vi "runBraking.vi"(6 "Fault?":bool, 7 "x acceleration":dbl, 8 "error in (no error)":errorcluster, 9 "Actuators in":T1, 10 "State in":T2, 11 "RunType in":refnum<class "RunType.lvclass">) -> (0 "error out":errorcluster, 1 "Actuators out":T1, 2 "State out":T2, 3 "RunType out":refnum<class "RunType.lvclass">)   [LabVIEW 2018, in "ControlLibrary.lvlib" / "RunType.lvclass"]
uses:
  RunType.lvclass
  TypeDef_ControlState.ctl
  TypeDef_DigitalOuts.ctl
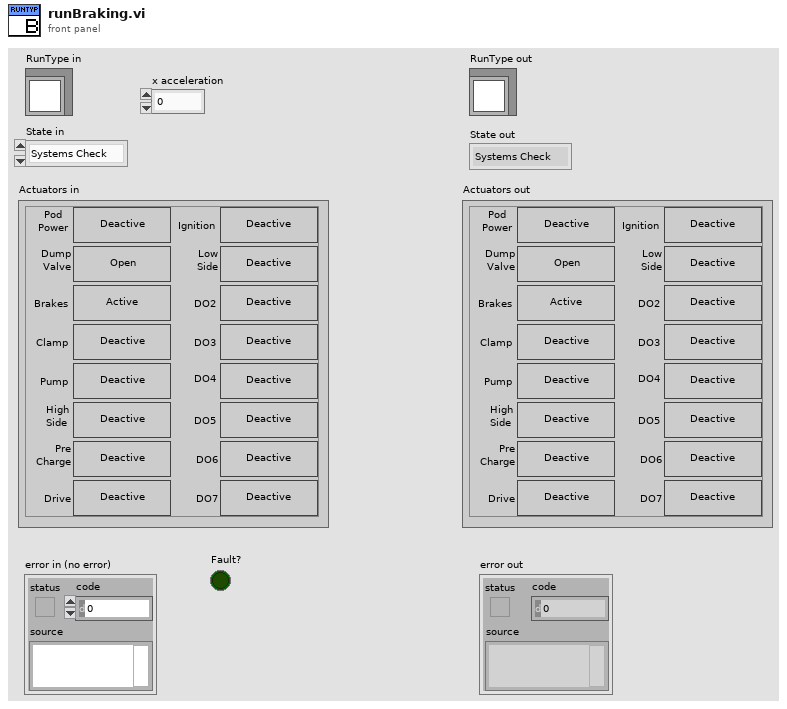
[diagram p1: front panel]
types:
  T1 = typedef "TypeDef_DigitalOuts.ctl" = cluster{"Pod Power":bool, "Dump Valve":bool, "Brakes":bool, "Clamp":bool, "Pump":bool, "Ignition":bool, "DO6":bool, "DO7":bool, "HighSide":bool, "Precharge":bool, "LowSide":bool, "DO3":bool, "DO4":bool, "DO5":bool, "DO62":bool, "DO72":bool}
  T2 = typedef "TypeDef_ControlState.ctl" = enum16{"Systems Check", "Idle", "Ready", "Pushing", "Coast", "Braking", "Fault", "Shutdown", "Service", "Precharge", "Blank"}
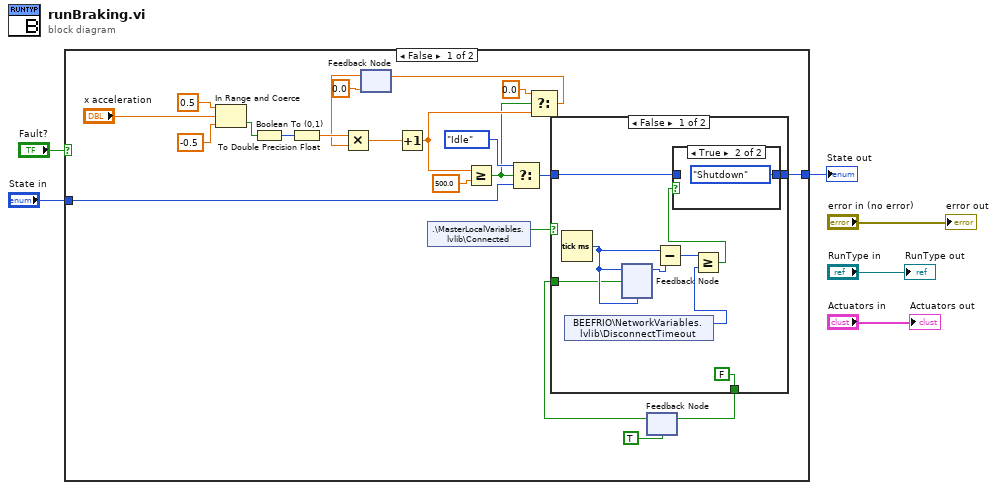
[diagram p0: block diagram]
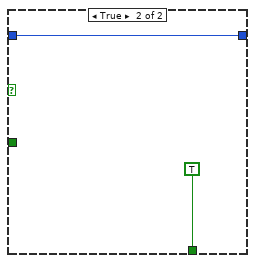
[diagram p3: hidden frame]
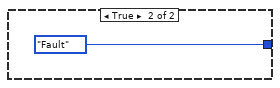
[diagram p4: hidden frame]
diagram:
  n1 = case shown="False" "Fault?" {
    tunnel: [w11 TypeDef_ControlState."Fault" ("State in")] -> w3
    tunnel: "State in" -> [w13 _]
    frame False {
      n2 = In Range and Coerce(upper limit=0.5, x="x acceleration", lower limit=-0.5) -> (In Range?=w19:bool)  [unwired: 1 out]
      n3 = Boolean To (0,1)(Boolean=w19) -> (0, 1=w23:i16)
      n4 = To Double Precision Float(number=w23) -> (double precision float=w28:dbl)
      n5 = feedback #1(0.0) -> (w21:dbl)
      n6 = Multiply(x=w28, y=w21) -> (x*y=w20:dbl)
      n7 = Increment(x=w20) -> (x+1=w25:dbl)
      n8 = shared-variable ".\\MasterLocalVariables.lvlib\\Connected"() -> (w12:bool)  [unwired: 1 in, 1 out]
      n9 = Greater Or Equal?(x=w25, y=500.0) -> (x >= y?=w15:bool)
      n10 = Select(t=TypeDef_ControlState."Idle" ("Enum"), s=w15, f=w13) -> (s? t:f=w10:T2)
      n11 = Select(t=0.0, s=w15, f=w25) -> (s? t:f=w26:dbl)
      n12 = feedback-in #1(w26) -> ()
      n13 = feedback #2(TRUE) -> (w7:bool)
      n14 = case shown="False" w12 {
        tunnel: [w37 w41] -> w11
        tunnel: w10 -> [w36 w41]
        tunnel: [FALSE TRUE] -> w8
        tunnel: w7 -> [w30 _]
        frame False {
          n15 = Tick Count (ms)() -> (millisecond timer value=w34:u32)
          n16 = shared-variable "BEEFRIO\\NetworkVariables.lvlib\\DisconnectTimeout"() -> (w29:u32)  [unwired: 1 in, 1 out]
          n17 = feedback #3(w34) -> (w35:u32)
          n18 = feedback-in #3(w34, w30) -> ()
          n19 = Subtract(x=w34, y=w35) -> (x-y=w33:u32)
          n20 = Greater Or Equal?(x=w33, y=w29) -> (x >= y?=w32:bool)
          n21 = case shown="True" w32 {
            tunnel: [w38 TypeDef_ControlState."Shutdown" ("State in")] -> w37
            tunnel: w36 -> [w38 _]
            frame False {
            }
            frame True {
            }
          }
        }
        frame True {
        }
      }
      n22 = feedback-in #2(w8) -> ()
    }
    frame True {
    }
  }
  "State out" <- w3
  "error out" <- "error in (no error)"
  "RunType out" <- "RunType in"
  "Actuators out" <- "Actuators in"
